vi "Set UUT Name.vi"(8 "error in":errorcluster, 11 "Base Software in":refnum<class "Main.lvclass">) -> (0 "error out":errorcluster, 3 "Base Software out":refnum<class "Main.lvclass">)   [LabVIEW 2023, in "Main.lvlib" / "Main.lvclass"]
uses:
  Project/Main.lvclass
  Custom Controls/g_Identifiers.vi
  Accessors/Indicators/Read UUT Name.vi
  builds/Tools/Chronometer.lvlibp/Chronometer Messages/Write UUT Msg/Write UUT Msg.lvclass
  builds/Engine/Engine.lvlibp/Project/Engine.lvclass
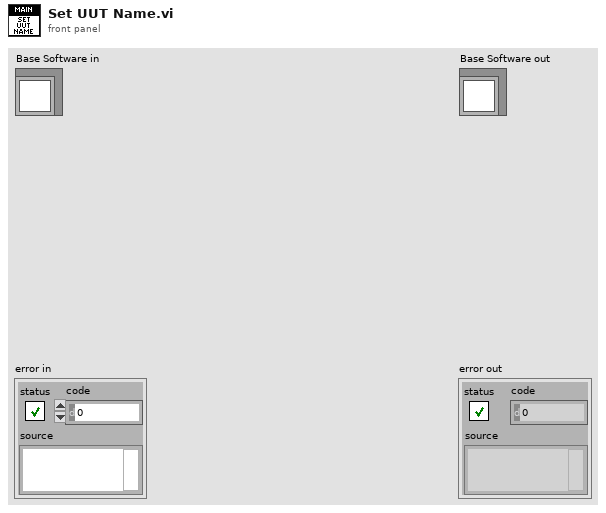
[diagram p1: front panel]
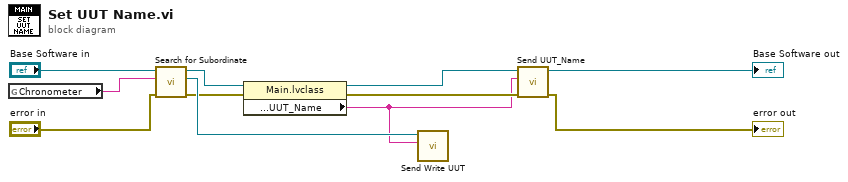
[diagram p0: block diagram]
diagram:
  n1 = global read "g_Identifiers.vi" "Chronometer"() -> (w10:string)
  n2 = call "Search for Subordinate.vi"("error in"="error in", "Identifier"=w10, "Base Software in"="Base Software in") -> ("error out"=w1:errorcluster, "Enqueuer"=w8:refnum<class "Message Enqueuer.lvclass">, "Base Software out"=w7:refnum<class "Main.lvclass">)  [unwired: 3 in, 3 out]
  n3 = property class="Main.lvclass"(reference=w7, error in=w1) -> (reference out=w6:refnum<class "Main.lvclass">, error out=w5:errorcluster, "Accessors:Indicators:UUT_Name"=w2:string)
  n4 = call "Send Write UUT.vi"("UUT"=w2, "Message Enqueuer"=w8) -> ()  [unwired: 8 in, 2 out]
  n5 = call "Send UUT_Name.vi"("error in"=w5, "UUT Name"=w2, "Engine in"=w6) -> ("error out"=→"error out":errorcluster, "Engine out"=→"Base Software out":refnum<class "Main.lvclass">)  [unwired: 7 in]
